vi "RS232C_WaitString_re.vi"(2 "Delimiter":string="\\r\\n", 3 "String to Receive":string, 4 "String to Send":string, 5 "PortNumber":i32) -> (0 "OK Done":bool, 1 "String Received":string)   [LabVIEW 2016]
panel:
  # "Port Number 0=COM1"
  # "Send the 'String to Send' to the Stage Controller and wait for the 'String to Receive'.\nAn Error occurs when received a different string or timed out."
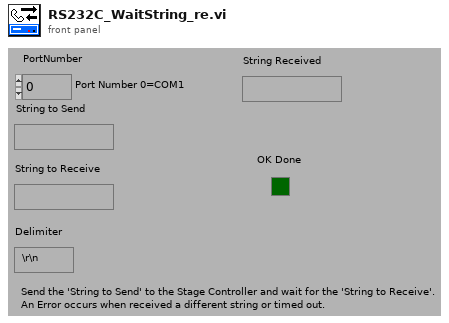
[diagram p1: front panel]
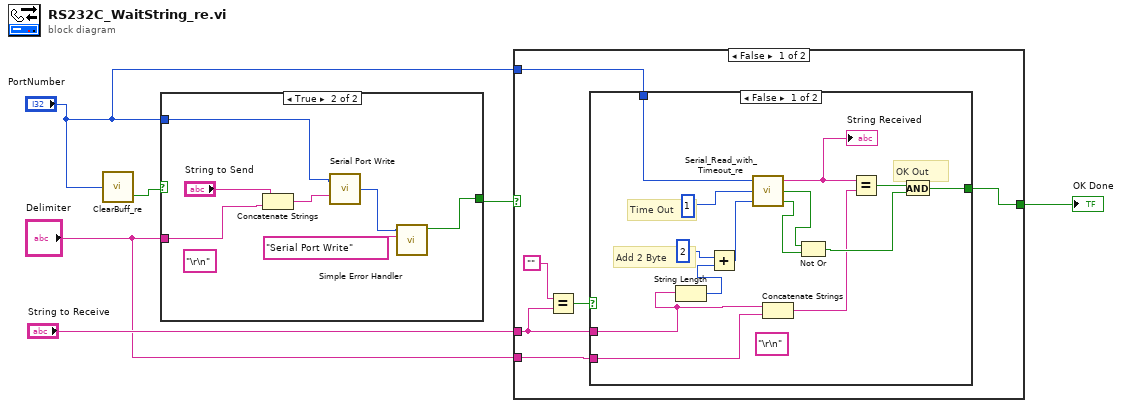
[diagram p0: block diagram]
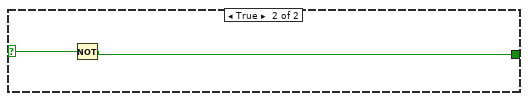
[diagram p3: hidden frame]
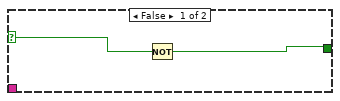
[diagram p4: hidden frame]
diagram:
  n1 = call "ClearBuff_re.vi"("PortNumber"="PortNumber") -> ("OK Done"=w6:bool)  [unwired: 1 out]
  n2 = case shown="True" w6 {
    selector: w6 -> [w8 _]
    tunnel: "PortNumber" -> [_ w10]
    tunnel: [w7 w11] -> w5
    tunnel: "Delimiter" -> [_ w9]
    frame False {
      n3 = Not(x=w8) -> (.not. x?=w7:bool)
    }
    frame True {
      (unwired) "\r\n"
      n4 = Concatenate Strings("String to Send", w9) -> (w14:string)
      n5 = call <vilib>:"Serial Port Write.vi"("string to write"=w14, "port number"=w10) -> ("error code"=w12:i32)
      n6 = call <vilib>:"Simple Error Handler.vi"("error code (no error:0)"=w12, "error source (\" \")"="Serial Port Write") -> ("error?"=w11:bool)  [unwired: 2 in, 5 out]
    }
  }
  n7 = case shown="False" w5 {
    selector: w5 -> [_ w38]
    tunnel: [w16 w37] -> w4
    tunnel: "String to Receive" -> [w17 _]
    tunnel: "PortNumber" -> [w19 _]
    tunnel: "Delimiter" -> [w18 _]
    frame False {
      n8 = Equal?(x="", y=w17) -> (x = y?=w20:bool)
      n9 = case shown="False" w20 {
        selector: w20 -> [_ w36]
        tunnel: [w30 w36] -> w16
        tunnel: w19 -> [w24 _]
        tunnel: w18 -> [w23 _]
        tunnel: w17 -> [w22 _]
        frame False {
          (unwired) "\r\n"
          # "OK Out"
          # "Time Out"
          # "Add 2 Byte"
          n10 = String Length(string=w22) -> (length=w28:i32)
          n11 = Add(x=2, y=w28) -> (x+y=w26:i32)
          n12 = call "Serial_Read_with_Timeout_re.vi"("Bytes to Read"=w26, "Timeout Limit"=1, "Port Number"=w24) -> ("Error Out"=w33:bool, "Timeout"=w34:bool, "Serial Read"=w29:string)
          "String Received" <- w29
          n13 = Concatenate Strings(w22, w23) -> (w25:string)
          n14 = Not Or(1:w33, 2:w34) -> (0:w31:bool)
          n15 = Equal?(x=w29, y=w25) -> (x = y?=w32:bool)
          n16 = And(x=w32, y=w31) -> (x .and. y?=w30:bool)
        }
        frame True {
        }
      }
    }
    frame True {
      n17 = Not(x=w38) -> (.not. x?=w37:bool)
    }
  }
  "OK Done" <- w4
